vi "读取csv.vi"() -> ()   [LabVIEW 2025]
uses:
  D:/LV test/LabVIEWConfigSecurity.dll
  LabVIEWConfigSecurity.dll
panel:
  out "第二个":string[](array[string])
  out "第一个":string[](array[string])
  out "机种名称":string[](array[string])
  out "Decrypt":string
  in  "对话框窗口（打开现有文件）":string
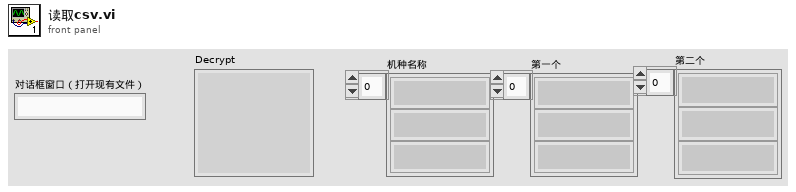
[diagram p1: front panel]
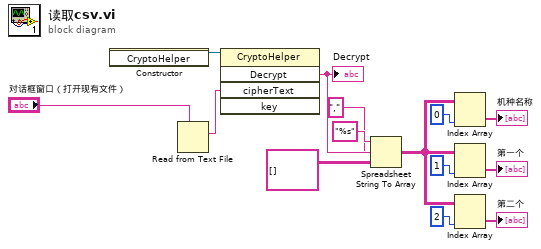
[diagram p0: block diagram]
diagram:
  n1 = constructor class="CryptoHelper"() -> (reference out=w14:refnum<k24>)  [unwired: 3 in, 2 out]
  n2 = Read from Text File(prompt (Open existing file)="对话框窗口（打开现有文件）") -> (text=w13:string)  [unwired: 3 in, 3 out]
  n3 = invoke on="调用节点" class="CryptoHelper" method="Decrypt"(reference=w14, "cipherText"=w13) -> ("Decrypt"=w11:string)  [unwired: 3 in, 4 out]
  "Decrypt" <- w11
  n4 = Spreadsheet String To Array(delimiter (Tab)="," ("分隔符(Tab)"), format string="%s" ("格式字符串"), spreadsheet string=w11, array type (2D Dbl)=string[][] []) -> (array=w7:string[][])
  n5 = Index Array(array=w7, index (col)=0 ("禁用的索引 (列)")) -> (element=→"机种名称":string[])  [unwired: 1 in]
  n6 = Index Array(array=w7, index (col)=1 ("禁用的索引 (列)")) -> (element=→"第一个":string[])  [unwired: 1 in]
  n7 = Index Array(array=w7, index (col)=2 ("禁用的索引 (列)")) -> (element=→"第二个":string[])  [unwired: 1 in]
